vi "sqrt (SubVI).vi"(6 "y":i32, 9 "x":i32, 10 "ym":dbl, 11 "xm":dbl) -> (3 "sq":dbl)   [LabVIEW 2018]
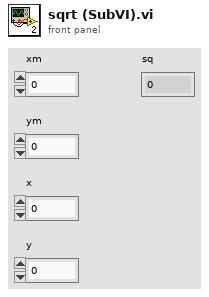
[diagram p1: front panel]
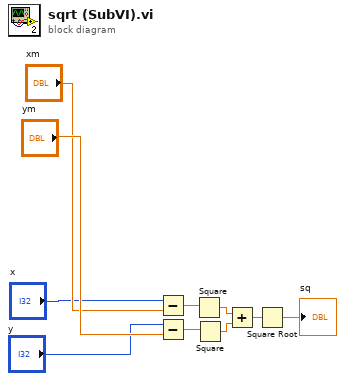
[diagram p0: block diagram]
diagram:
  n1 = Subtract(x="x", y="xm") -> (x-y=w5:dbl)
  n2 = Subtract(x="y", y="ym") -> (x-y=w6:dbl)
  n3 = Square(x=w5) -> (x^2=w7:dbl)
  n4 = Square(x=w6) -> (x^2=w8:dbl)
  n5 = Add(x=w7, y=w8) -> (x+y=w9:dbl)
  n6 = Square Root(x=w9) -> (sqrt(x)=→"sq":dbl)
